vi "Bin Flush Data to Log File.vi"(8 "error in (no error)":errorcluster, 10 "Data Queue":refnum<queue>, 11 "Logging Configuration":T1) -> (0 "error out":errorcluster)   [LabVIEW 2017, in "Logging.lvlib"]
uses:
  Logging.lvlib
  Logging Configuration.ctl
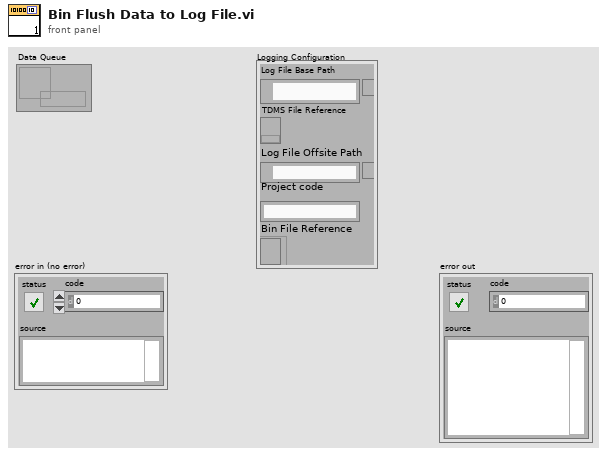
[diagram p1: front panel]
types:
  T1 = typedef "Logging.lvlib/Logging Configuration.ctl" = cluster{"Log File Base Path":path, "TDMS File Reference":refnum<k34>, "Log File Offsite Path":path, "Project code":string, "Bin File Reference":refnum<file>}
  T2 = enum16{"big-endian, network order", "native, host order", "little-endian"}
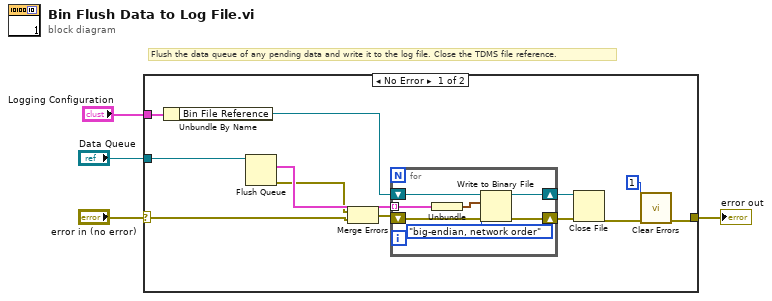
[diagram p0: block diagram]
diagram:
  # "Flush the data queue of any pending data and write it to the log file. Close the TDMS file reference."
  n1 = case shown="No Error" "error in (no error)" {
    selector: "error in (no error)" -> [w14 w24]
    tunnel: "Data Queue" -> [w10 _]
    tunnel: "Logging Configuration" -> [w12 _]
    tunnel: [w5 w24] -> w2
    frame No Error {
      n2 = Unbundle By Name(w12) -> ("Bin File Reference"=w11:refnum<file>)
      n3 = Flush Queue(queue=w10) -> (remaining elements=w16:cluster{"Array":waveform(dbl)[]}[], error out=w8:errorcluster)  [unwired: 1 in, 1 out]
      n4 = Merge Errors(w8, w14) -> (w13:errorcluster)
      n5 = for {
        shift-right: [w20] -> w15
        shift-left: w11 -> [w21]
        shift-right: [w22] -> w7
        shift-left: w13 -> [w23]
        tunnel: w16 -> [w19] mode=indexing
        n6 = Unbundle(w19) -> ("Array"=w17:waveform(dbl)[])
        n7 = Write to Binary File(file (use dialog)=w21, data=w17, error in=w23, 9:T2."big-endian, network order" ("byte order (0:big-endian, network order)")) -> (refnum out=w20:refnum<file>, error out=w22:errorcluster)  [unwired: 2 in, 1 out]
      }
      n8 = Close File(refnum=w15, error in=w7) -> (error out=w6:errorcluster)  [unwired: 1 out]
      n9 = call <vilib>:"Clear Errors.vi"("error in (no error)"=w6, "specific error code to clear (0: all)"=1) -> ("error out"=w5:errorcluster)  [unwired: 4 in, 1 out]
    }
    frame Error {
    }
  }
  "error out" <- w2
